vi "New motor Control integrated remodeled state based with PID.vi"(2 "Error in":errorcluster, 3 "Yaw":dbl, 4 "States":T2) -> (0 "Error out":errorcluster, 1 "Speed and distance cluster":T1)   [LabVIEW 2018]
uses:
  Motor Control/States for motor control.ctl
  <vilib>/addons/control/pid/pid.llb/PID (DBL).vi
  <vilib>/addons/control/pid/NI_PID_pid.lvlib
panel:
  out "Output":cluster{dbl, dbl, dbl}
  in  "Boolean":bool=TRUE
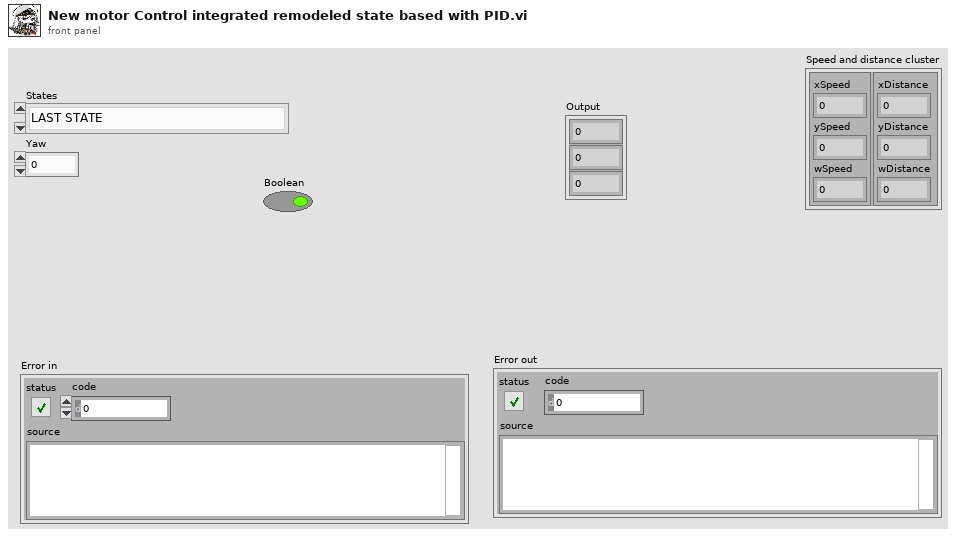
[diagram p1: front panel]
types:
  T1 = cluster{cluster{"xSpeed":dbl, "ySpeed":dbl, "wSpeed":dbl}, cluster{"xDistance":dbl, "yDistance":dbl, "wDistance":dbl}}
  T2 = typedef "States for motor control.ctl" = enum16{"LAST STATE", "STOP", "FORWARD", "BACKWARD", "LEFT", "RIGHT", "RCW", "ACW", "INIT", "RESET ENCODERS"}
  T3 = cluster{"Encoder 0":dbl, "Encoder 1":dbl, "Encoder 2":dbl}
  T4 = cluster{"xTargetSpeed":dbl, "yTargetSpeed":dbl, "wTargetSpeed":dbl}
  T5 = cluster{"proportional gain (Kc)":dbl, "integral time (Ti, min)":dbl, "derivative time (Td, min)":dbl}
  T6 = cluster{"Distance M0 ":dbl, "Distance M1 ":dbl, "Distance M2 ":dbl}
  T7 = cluster{"xDistance":dbl, "yDistance":dbl, "wDistance":dbl}
  T8 = cluster{"xSpeed":dbl, "ySpeed":dbl, "wSpeed":dbl}
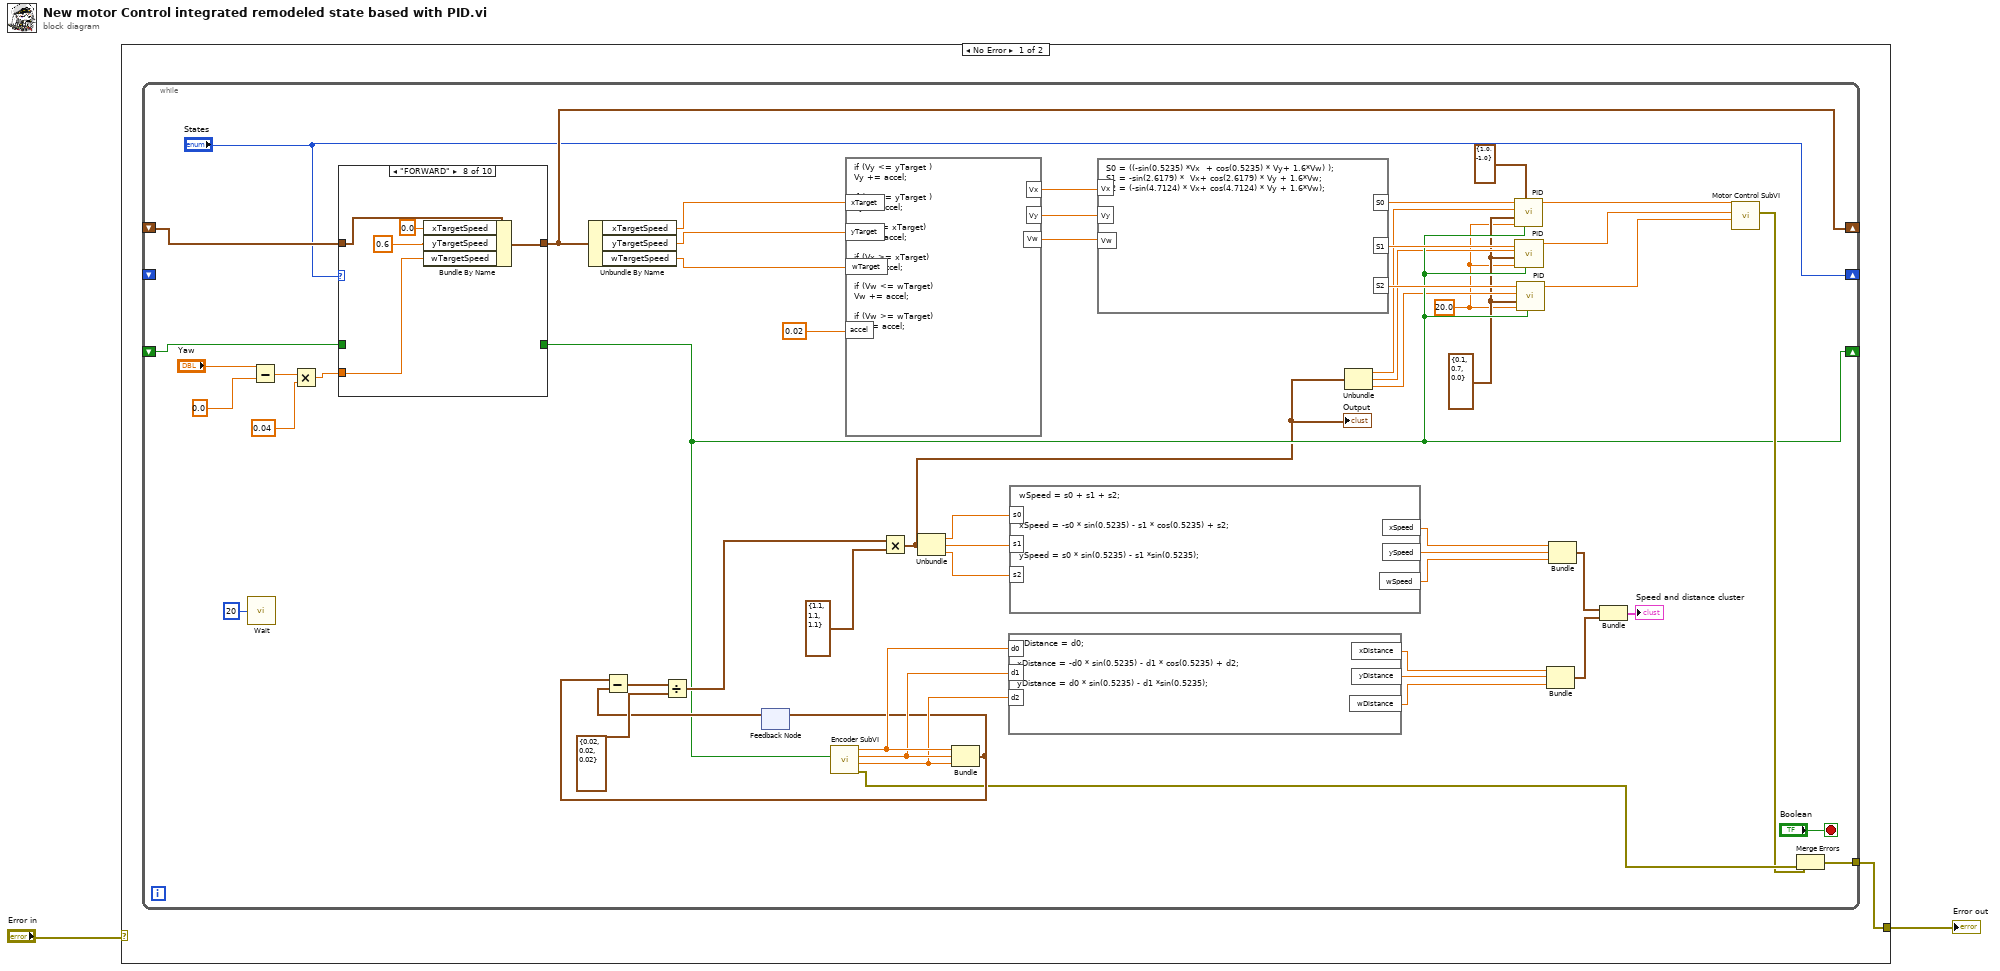
[diagram p0: block diagram]
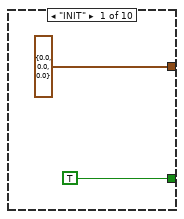
[diagram p2: hidden frame]
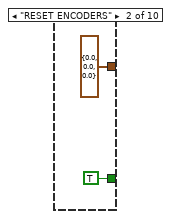
[diagram p3: hidden frame]
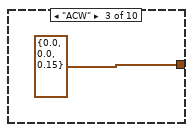
[diagram p4: hidden frame]
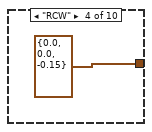
[diagram p5: hidden frame]
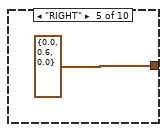
[diagram p6: hidden frame]
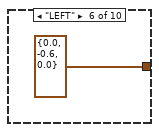
[diagram p7: hidden frame]
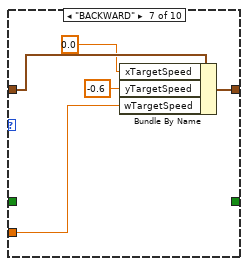
[diagram p8: hidden frame]
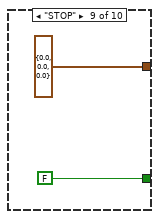
[diagram p9: hidden frame]
diagram:
  n1 = case shown="No Error" "Error in" {
    selector: "Error in" -> [_ w81]
    tunnel: [w3 w81] -> w1
    frame No Error {
      n2 = while {
        shift-right: [w40] -> _
        shift-left: _ -> [w39]
        tunnel: [w34] -> w3
        shift-right: [w11] -> _
        shift-left: _ -> [w33]
        shift-right: ["States"] -> _
        shift-left: _ -> [_]
        stop <- "Boolean" stop-if-true
        w5 = 20.0 ("dt (s)")
        w6 = T5 {"proportional gain (Kc)"=0.1, "integral time (Ti, min)"=0.7, "derivative time (Td, min)"=0.0} ("PID gains")
        n3 = call "Wait"("Count(uSec)"=u32 20) -> ()  [unwired: 1 out]
        n4 = Subtract(x="Yaw", y=0.0) -> (x-y=w22:dbl)
        n5 = Multiply(x=w22, y=0.04) -> (x*y=w20:dbl)
        n6 = case shown="\"FORWARD\"" "States" {
          tunnel: [T4 {"xTargetSpeed"=0.0, "yTargetSpeed"=0.0, "wTargetSpeed"=0.0} ("Target Speed") T4 {"xTargetSpeed"=0.0, "yTargetSpeed"=0.0, "wTargetSpeed"=0.0} ("Target Speed") T4 {"xTargetSpeed"=0.0, "yTargetSpeed"=0.0, "wTargetSpeed"=0.15} ("Target Speed") T4 {"xTargetSpeed"=0.0, "yTargetSpeed"=0.0, "wTargetSpeed"=-0.15} ("Target Speed") T4 {"xTargetSpeed"=0.0, "yTargetSpeed"=0.6, "wTargetSpeed"=0.0} ("Target Speed") T4 {"xTargetSpeed"=0.0, "yTargetSpeed"=-0.6, "wTargetSpeed"=0.0} ("Target Speed") w72 w75 T4 {"xTargetSpeed"=0.0, "yTargetSpeed"=0.0, "wTargetSpeed"=0.0} ("Target Speed") w80] -> w40
          tunnel: w39 -> [_ _ _ _ _ _ w71 w76 _ w80]
          tunnel: [TRUE ("Reset Encoders") TRUE ("Reset Encoders") _ _ _ _ _ _ FALSE ("Reset Encoders") _] -> w11
          tunnel: w33 -> [_ _ _ _ _ _ _ _ _ _]
          tunnel: w20 -> [_ _ _ _ _ _ w68 w77 _ _]
          frame "INIT" {
          }
          frame "RESET ENCODERS" {
          }
          frame "ACW" {
          }
          frame "RCW" {
          }
          frame "RIGHT" {
          }
          frame "LEFT" {
          }
          frame "BACKWARD" {
            n7 = Bundle By Name(cluster=w71, "xTargetSpeed"=0.0, "yTargetSpeed"=-0.6, "wTargetSpeed"=w68) -> (w72:T4)
          }
          frame "FORWARD" {
            n8 = Bundle By Name(cluster=w76, "xTargetSpeed"=0.0, "yTargetSpeed"=0.6, "wTargetSpeed"=w77) -> (w75:T4)
          }
          frame "STOP" {
          }
          frame "LAST STATE" {
          }
        }
        n9 = Unbundle By Name(w40) -> ("xTargetSpeed"=w27:dbl, "yTargetSpeed"=w26:dbl, "wTargetSpeed"=w25:dbl)
        n10 = feedback #1() -> (w52:T6)  [unwired: 1 in]
        n11 = call "Encoder SubVI.vi"("Reset Encoders"=w11) -> ("error out"=w36:errorcluster, "Distance M2"=w49:dbl, "Distance M1"=w50:dbl, "Distance M0"=w51:dbl)  [unwired: 7 in]
        n12 = formula code="if (Vy <= yTarget )\nVy += accel;\n\nif (Vy >= yTarget )\nVy -= accel;\n\nif(Vx <= xTarget)\nVx += accel;\n\nif (Vx >= xTarget)\nVx -= accel;\n\nif (Vw <= wTarget)\nVw += accel;\n\nif (Vw >= wTarget)\nVw -= accel;"("xTarget"=w27, "yTarget"=w26, "wTarget"=w25, "accel"=0.02 ("input variable")) -> ("Vy"=w30:dbl, "Vx"=w31:dbl, "Vw"=w29:dbl)
        n13 = Bundle("Distance M0"=w51, "Distance M1"=w50, "Distance M2"=w49) -> (w41:T6)  [unwired: 1 in]
        n14 = Subtract(x=w41, y=w52) -> (x-y=w59:T6)
        n15 = Divide(x=w59, y=T3 {"Encoder 0"=0.02, "Encoder 1"=0.02, "Encoder 2"=0.02}) -> (x/y=w45:cluster{dbl, dbl, dbl})
        n16 = feedback-in #1(w41) -> ()
        n17 = Multiply(x=w45, y=cluster{dbl, dbl, dbl} {1.1, 1.1, 1.1}) -> (x*y=w10:cluster{dbl, dbl, dbl})
        "Output" <- w10
        n18 = Unbundle(w10) -> (w43:dbl, w54:dbl, w53:dbl)
        n19 = formula code="wDistance = d0;\n\nxDistance = -d0 * sin(0.5235) - d1 * cos(0.5235) + d2;\n\nyDistance = d0 * sin(0.5235) - d1 *sin(0.5235);"("d0"=w51, "d1"=w50, "d2"=w49) -> ("xDistance"=w48:dbl, "wDistance"=w46:dbl, "yDistance"=w47:dbl)
        n20 = formula code="wSpeed = s0 + s1 + s2;\n\n\nxSpeed = -s0 * sin(0.5235) - s1 * cos(0.5235) + s2;\n\n\nySpeed = s0 * sin(0.5235) - s1 *sin(0.5235);"("s0"=w43, "s1"=w54, "s2"=w53) -> ("xSpeed"=w56:dbl, "ySpeed"=w57:dbl, "wSpeed"=w55:dbl)
        n21 = formula code="S0 = ((-sin(0.5235) *Vx  + cos(0.5235) * Vy+ 1.6*Vw) );\nS1 = -sin(2.6179) *  Vx+ cos(2.6179) * Vy + 1.6*Vw;\nS2 = (-sin(4.7124) * Vx+ cos(4.7124) * Vy + 1.6*Vw);"("Vx"=w31, "Vy"=w30, "Vw"=w29) -> ("S0"=w18:dbl, "S1"=w17:dbl, "S2"=w16:dbl)
        n22 = Unbundle(w10) -> (w9:dbl, w8:dbl, w7:dbl)
        n23 = call-poly <vilib>:"PID.vi"("reinitialize? (F)"=w11, "output range"=cluster{"output high":dbl, "output low":dbl} {"output high"=1.0, "output low"=-1.0}, "dt (s)"=w5, "PID gains"=w6, "process variable"=w9, "setpoint"=w18) -> ("output"=w15:dbl)  [unwired: 4 in, 1 out]
        n24 = call-poly <vilib>:"PID.vi"("reinitialize? (F)"=w11, "dt (s)"=w5, "PID gains"=w6, "process variable"=w8, "setpoint"=w17) -> ("output"=w14:dbl)  [unwired: 5 in, 1 out]
        n25 = call-poly <vilib>:"PID.vi"("reinitialize? (F)"=w11, "dt (s)"=w5, "PID gains"=w6, "process variable"=w7, "setpoint"=w16) -> ("output"=w13:dbl)  [unwired: 5 in, 1 out]
        n26 = Bundle("xDistance"=w48, "yDistance"=w47, "wDistance"=w46) -> (w38:T7)  [unwired: 1 in]
        n27 = Bundle("xSpeed"=w56, "ySpeed"=w57, "wSpeed"=w55) -> (w32:T8)  [unwired: 1 in]
        n28 = Bundle(w32, w38) -> (→"Speed and distance cluster":T1)  [unwired: 1 in]
        n29 = call "Motor Control SubVI.vi"("Speed M2"=w13, "Speed M1"=w14, "Speed M0"=w15) -> ("Motor Error"=w35:errorcluster)  [unwired: 8 in]
        n30 = Merge Errors(w35, w36) -> (w34:errorcluster)
      }
    }
    frame Error {
    }
  }
  "Error out" <- w1
